vi "ErrorHandling.checkForErrorAndHandle.vi"(8 "error in (no error)":errorcluster, 9 "StopOnError":bool, 10 "Comment":string, 11 "ErrorHandling in":refnum<data-value>) -> (0 "error out":errorcluster, 1 "Stop":bool, 3 "ErrorHandling out":refnum<data-value>)   [LabVIEW 2016, in "ErrorHandling.lvclass"]
doc: "Erfasst einen Error, sucht sich allfällige Custom-Errors heraus\n\n15.04.14/ sige"
uses:
  ErrorHandling.lvclass
  ErrorHandling.lvclass/ErrorHandling.ctl
  ErrorHandling.OccurredErrorDataStruct.ctl
  <vilib>/dlg_ctls.llb/Space Constant.vi
  <vilib>/Utility/error.llb/Search and Replace Pattern.vi
  <vilib>/Utility/error.llb/Trim Whitespace.vi
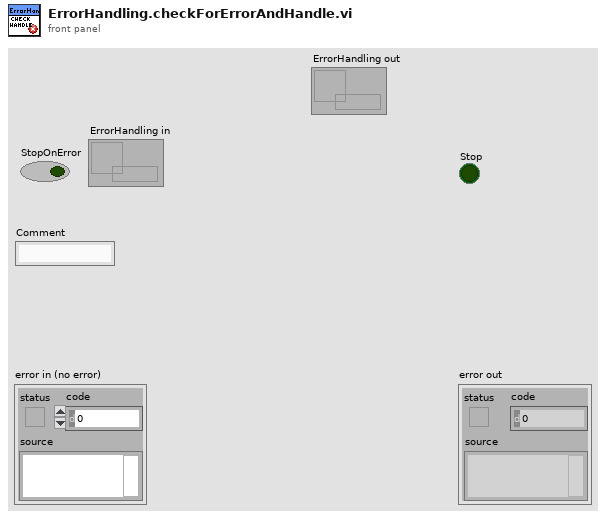
[diagram p1: front panel]
types:
  T1 = typedef "ErrorHandling.lvclass/ErrorHandling.OccurredErrorDataStruct.ctl" = cluster{"Error":errorcluster, "Caller":string, "Comment":string, "Timestamp":timestamp, "Stopped":bool, "ErrorCusterString":string, "ErrorIndex":u64}
  T2 = cluster{"LVError":errorcluster, "Action":enum16{"continue", "stop"}, "Source":string}[]
  T3 = cluster{"LVError":errorcluster, "Action":enum16{"continue", "stop"}, "Source":string}
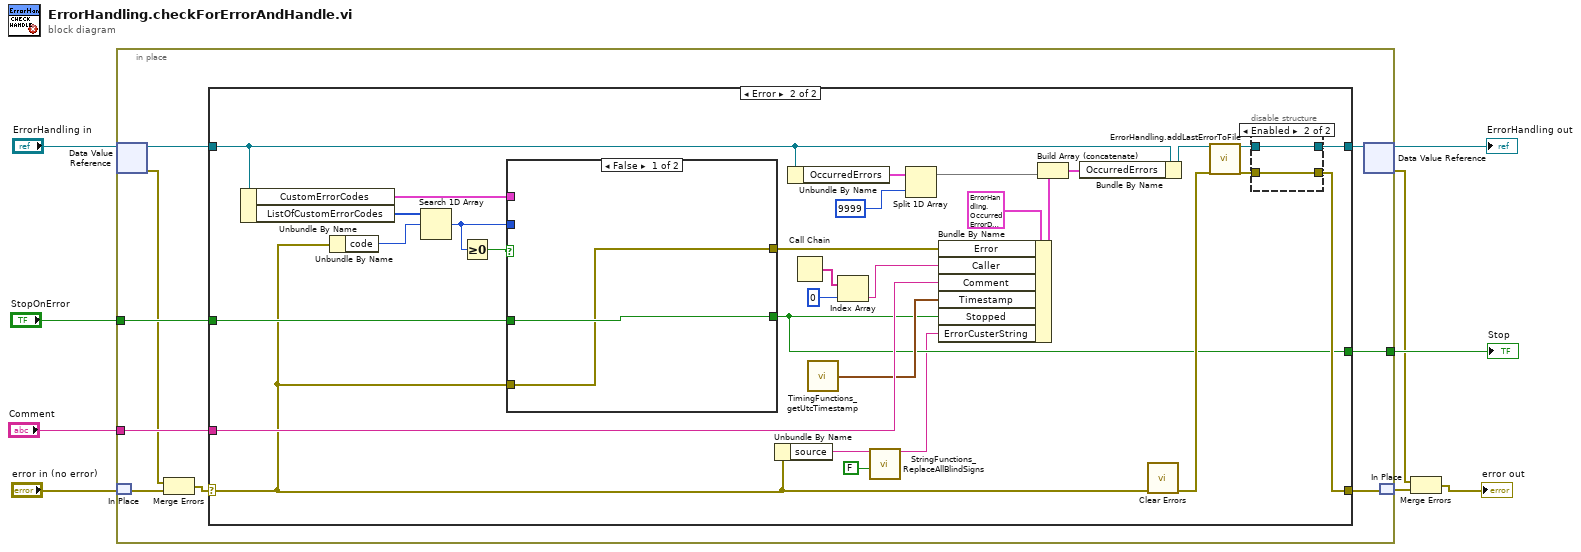
[diagram p0: block diagram]
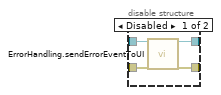
[diagram p3: hidden frame]
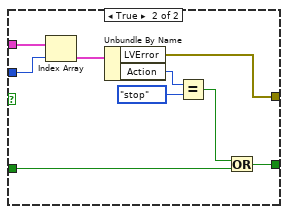
[diagram p4: hidden frame]
diagram:
  n1 = in-place {
    in-place-border: "StopOnError" -> [w18]
    in-place-border: "Comment" -> [w17]
    in-place-border: [w16] -> w7
    n2 = in-place-dvr #1("ErrorHandling in") -> (w15:refnum<class "ErrorHandling.lvclass">, w11:errorcluster)
    n3 = in-place-match #2("error in (no error)") -> (w12:errorcluster)
    n4 = Merge Errors(w11, w12) -> (w10:errorcluster)
    n5 = case shown="Error" w10 {
      selector: w10 -> [w19 w25]
      tunnel: [w19 w28] -> w13
      tunnel: [w20 w29] -> w14
      tunnel: w15 -> [w20 w44]
      tunnel: w18 -> [_ w45]
      tunnel: w17 -> [_ w36]
      tunnel: [_ w24] -> w16
      frame No Error {
        # "Siehe Error-Case"
      }
      frame Error {
        n6 = Unbundle By Name(w44) -> ("CustomErrorCodes"=w47:T2, "ListOfCustomErrorCodes"=w50:i32[])
        n7 = Unbundle By Name(w25) -> ("code"=w49:i32)
        n8 = Search 1D Array(1D array=w50, element=w49) -> (index of element=w46:i32)  [unwired: 1 in]
        n9 = Greater Or Equal To 0?(x=w46) -> (x >= 0?=w48:bool)
        n10 = case shown="False" w48 {
          tunnel: w47 -> [_ w67]
          tunnel: w46 -> [_ w66]
          tunnel: w45 -> [w58 w61]
          tunnel: [w58 w60] -> w24
          tunnel: [w57 w59] -> w38
          tunnel: w25 -> [w57 _]
          frame False {
          }
          frame True {
            n11 = Index Array(array=w67, index=w66) -> (element=w65:T3)
            n12 = Unbundle By Name(w65) -> ("LVError"=w59:errorcluster, "Action"=w64:enum16{"continue", "stop"})
            n13 = Equal?(x=w64, y=enum16{"continue", "stop"}."stop") -> (x = y?=w62:bool)
            n14 = Or(x=w62, y=w61) -> (x .or. y?=w60:bool)
          }
        }
        n15 = Unbundle By Name(w25) -> ("source"=w23:string)
        n16 = Unbundle By Name(w44) -> ("OccurredErrors"=w43:T1[])
        n17 = Call Chain() -> (call chain=w41:string[])
        n18 = call "TimingFunctions_getUtcTimestamp.vi"() -> ("UTC-time"=w35:timestamp)  [unwired: 1 in]
        n19 = Index Array(array=w41, index=0) -> (element=w37:string)
        n20 = call "StringFunctions_ReplaceAllBlindSigns.vi"("String"=w23, "RemoveSpaceAswell"=FALSE) -> ("ModifiedString"=w22:string)  [unwired: 16 in, 1 out]
        n21 = Split 1D Array(array=w43, index=9999) -> (first subarray=w27:T1[])  [unwired: 1 out]
        n22 = Bundle By Name(cluster=T1 {"Error"={"status"=FALSE, "code"=0, "source"=""}, "Caller"="", "Comment"="", "Timestamp"=timestamp(0 s since 1904-01-01), "Stopped"=FALSE, "ErrorCusterString"="", "ErrorIndex"=0} ("Cluster"), "Error"=w38, "Caller"=w37, "Comment"=w36, "Timestamp"=w35, "Stopped"=w24, "ErrorCusterString"=w22) -> (w34:T1)
        n23 = Build Array (concatenate)(w34, w27) -> (w42:T1[])
        n24 = Bundle By Name(cluster=w44, "OccurredErrors"=w42) -> (w33:refnum<class "ErrorHandling.lvclass">)
        n25 = call <vilib>:"Clear Errors.vi"("error in (no error)"=w25) -> ("error out"=w32:errorcluster)  [unwired: 5 in, 1 out]
        n26 = call "ErrorHandling.addLastErrorToFile.vi"("ErrorHandling in"=w33, "error in (no error)"=w32) -> ("ErrorHandling out"=w30:refnum<class "ErrorHandling.lvclass">, "error out"=w31:errorcluster)  [unwired: 16 in]
        n27 = disable-structure shown="Enabled" {
          disable-tunnel: w31 -> [w54 w56]
          disable-tunnel: w30 -> [w53 w55]
          disable-tunnel: [w52 w55] -> w29
          disable-tunnel: [w51 w56] -> w28
          frame Disabled {
            n28 = call "ErrorHandling.sendErrorEventToUI.vi"("ErrorHandling in"=w53, "error in (no error)"=w54) -> ("ErrorHandling out"=w52:refnum<class "ErrorHandling.lvclass">, "error out"=w51:errorcluster)  [unwired: 16 in]
          }
          frame Enabled {
          }
        }
      }
    }
    n29 = in-place-dvr #1(w14) -> (→"ErrorHandling out":refnum<data-value>, w1:errorcluster)
    n30 = in-place-match #2(w13) -> (w2:errorcluster)
  }
  "Stop" <- w7
  n31 = Merge Errors(w1, w2) -> (→"error out":errorcluster)
